vi "tipos de dados.vi"() -> ()   [LabVIEW 2018]
panel:
  out "String 2":string
  in  "String":string
  out "Array 2":dbl[](array[numeric])
  in  "Array":dbl[](array[numeric])
  out "Boolean 2":bool
  in  "Boolean":bool
  out "decimal out":dbl
  out "inteiro out":i32
  in  "decimal 2":dbl
  in  "inteiro":i32
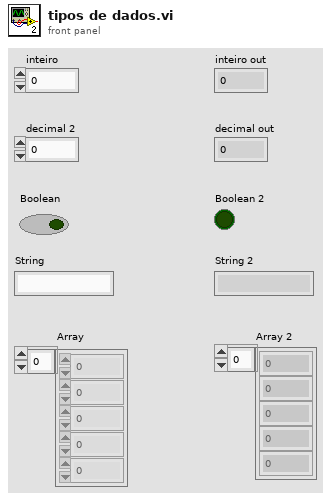
[diagram p1: front panel]
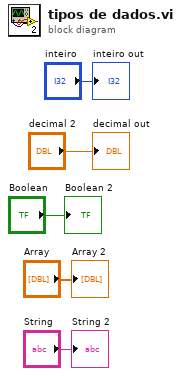
[diagram p0: block diagram]
diagram:
  "inteiro out" <- "inteiro"
  "decimal out" <- "decimal 2"
  "Boolean 2" <- "Boolean"
  "Array 2" <- "Array"
  "String 2" <- "String"
